vi "Shutdown Master.vi"(8 "error in (no error)":errorcluster, 11 "network master in":refnum<class "Network Master.lvclass">) -> (0 "error out":errorcluster, 3 "network master out":refnum<class "Network Master.lvclass">)   [LabVIEW 2017, in "SubVIs.lvlib" / "Network Master.lvclass"]
doc: "This provides an interface for the master to close a connection to the slave."
uses:
  <vilib>/Modbus/subvis/Protocol/Interfaces/Network Master/Network Master.lvclass
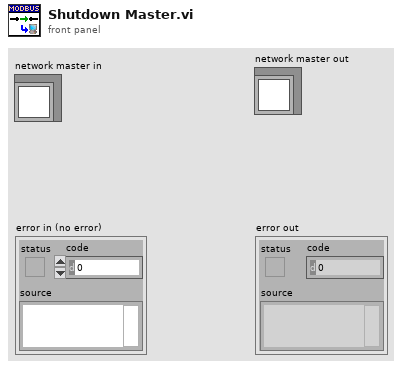
[diagram p1: front panel]
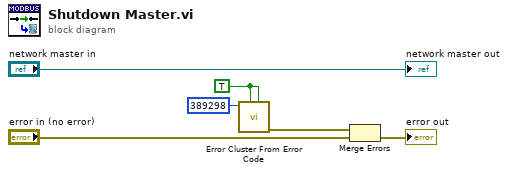
[diagram p0: block diagram]
diagram:
  w1 = TRUE ("show call chain? (False)")
  n1 = call <vilib>:"Error Cluster From Error Code.vi"("is warning? (False)"=w1, "show call chain? (False)"=w1, "error code (0)"=389298) -> ("error out"=w3:errorcluster)  [unwired: 6 in]
  n2 = Merge Errors(w3, "error in (no error)") -> (→"error out":errorcluster)
  "network master out" <- "network master in"
